vi "_Test Generate Coverage Table.vi"(8 "error in (no error)":errorcluster, 11 "Test Case In":refnum<class "Coverage Test.lvclass">) -> (0 "error out":errorcluster, 3 "Test Case Out":refnum<class "Coverage Test.lvclass">)   [LabVIEW 2020, in "LUnit Tests.lvlib" / "Coverage Test.lvclass"]
uses:
  Coverage Test.lvclass
  Coverage Test.lvclass/Coverage Test.ctl
  01074fa8-ee8a-411d-bc8b-fc92c4f90959.vi
  source/Framework/Coverage Analyzer/Coverage Analyzer.lvclass
  source/Framework/Coverage Analyzer Result View/Coverage Analyzer Result View.lvclass
  source/Framework/Coverage Analyzer Result View/Coverage Analyzer View Data.ctl
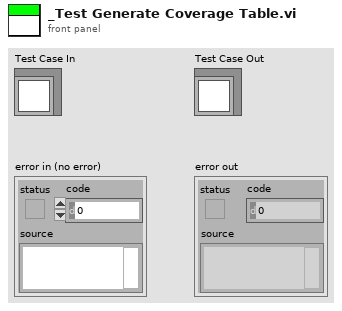
[diagram p1: front panel]
types:
  T1 = typedef "Coverage Analyzer Result View.lvclass/Coverage Analyzer View Data.ctl" = cluster{"Code Coverage":map{path, dbl}}
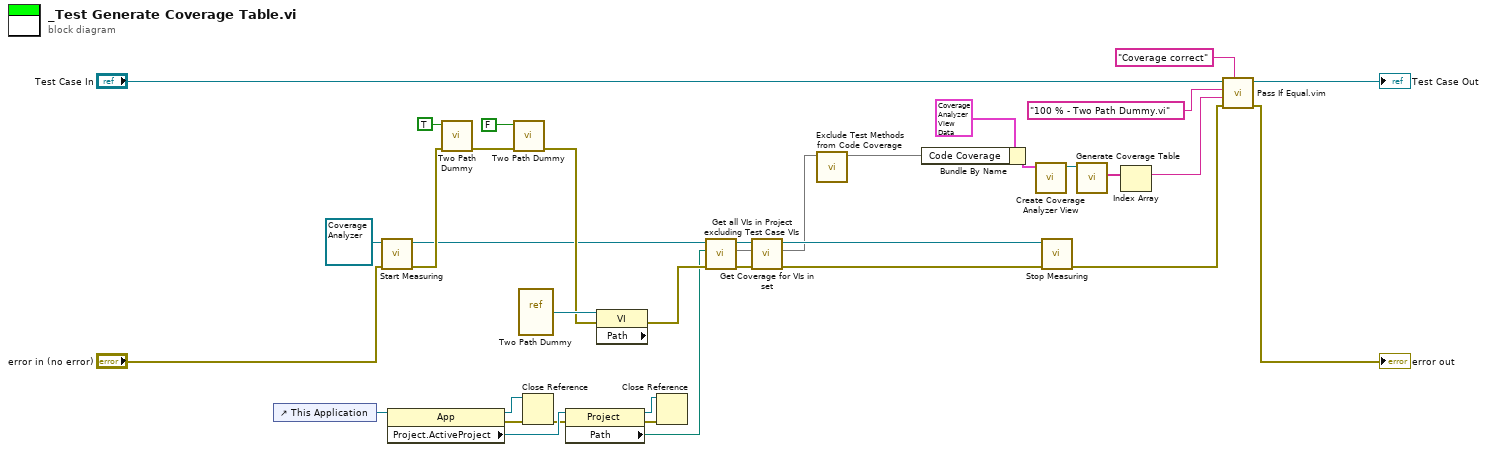
[diagram p0: block diagram]
diagram:
  n1 = control-ref of="This Application"() -> (w19:refnum<vi>)
  n2 = call "Start Measuring.vi"("error in (no error)"="error in (no error)", "Coverage Analyzer in"=refnum<class "Coverage Analyzer.lvclass"> refnum) -> ("error out"=w28:errorcluster, "Coverage Analyzer out"=w4:refnum<class "Coverage Analyzer.lvclass">)  [unwired: 8 in]
  n3 = property class="App"(reference=w19) -> (reference out=w14:refnum<vi>, error out=w11:errorcluster, "Project.ActiveProject"=w18:refnum<vi>)  [unwired: 1 in]
  n4 = call "Two Path Dummy.vi"("error in (no error)"=w28, "Boolean"=TRUE) -> ("error out"=w32:errorcluster)  [unwired: 9 in]
  n5 = call "Two Path Dummy.vi"("error in (no error)"=w32, "Boolean"=FALSE) -> ("error out"=w23:errorcluster)  [unwired: 9 in]
  n6 = vi-ref "Two Path Dummy.vi"() -> (w34:refnum<vi>)
  n7 = Close Reference(reference=w14, error in (no error)=w11) -> (error out=w10:errorcluster)
  n8 = property class="Project"(reference=w18, error in=w10) -> (reference out=w13:refnum<vi>, error out=w12:errorcluster, "Path"=w1:path)
  n9 = property class="VI" props=["Path"](reference=w34, error in=w23) -> (error out=w24:errorcluster)  [unwired: 2 out]
  n10 = Close Reference(reference=w13, error in (no error)=w12) -> ()  [unwired: 1 out]
  n11 = call "Get all VIs in Project excluding Test Case VIs.vi"("error in (no error)"=w24, "Path"=w1, "Coverage Analyzer in"=w4) -> ("error out"=w5:errorcluster, "VIs"=w2:set{path}, "Coverage Analyzer out"=w3:refnum<class "Coverage Analyzer.lvclass">)  [unwired: 6 in]
  n12 = call "Get Coverage for VIs in set.vi"("error in (no error)"=w5, "VIs"=w2, "Coverage Analyzer in"=w3) -> ("error out"=w20:errorcluster, "Code Coverage"=w16:map{path, dbl}, "Coverage Analyzer out"=w21:refnum<class "Coverage Analyzer.lvclass">)  [unwired: 6 in]
  n13 = call "Exclude Test Methods from Code Coverage.vi"("Code Coverage"=w16) -> ("Filtered Code Coverage"=w15:map{path, dbl})  [unwired: 10 in]
  n14 = Bundle By Name(cluster=T1 {"Code Coverage"={}} ("Data"), "Code Coverage"=w15) -> (w7:T1)
  n15 = call "Create Coverage Analyzer View.vi"("Coverage Analyzer Result View in"=w7) -> ("Coverage Analyzer Result View out"=w6:refnum<class "Coverage Analyzer Result View.lvclass">)  [unwired: 9 in, 1 out]
  n16 = call "Stop Measuring.vi"("error in (no error)"=w20, "Coverage Analyzer in"=w21) -> ("error out"=w26:errorcluster)  [unwired: 8 in, 1 out]
  n17 = call "Generate Coverage Table.vi"("Coverage Analyzer Result View In"=w6) -> ("Item Names"=w8:string[])  [unwired: 8 in, 2 out]
  n18 = Index Array(array=w8) -> (element=w9:string)  [unwired: 1 in]
  n19 = call "Pass If Equal.vim"("Description"="Coverage correct", "error in (no error)"=w26, "Actual"=w9, "Expected"="100 % - Two Path Dummy.vi" ("String"), "LUnit Test Case In"="Test Case In") -> ("error out"=→"error out":errorcluster, "LUnit Test Case Out"=→"Test Case Out":refnum<class "Coverage Test.lvclass">)  [unwired: 5 in]
